vi "remove specific file path.vi"(8 "error in":errorcluster, 10 "Path":path, 11 "VI modification collection in":refnum<class "VI modification collection.lvclass">) -> (0 "error out":errorcluster, 3 "VI modification collection out":refnum<class "VI modification collection.lvclass">)   [LabVIEW 2013, in "VI modification collection.lvclass"]
uses:
  VI modification collection.lvclass
  VI modification collection.lvclass/VI modification collection.ctl
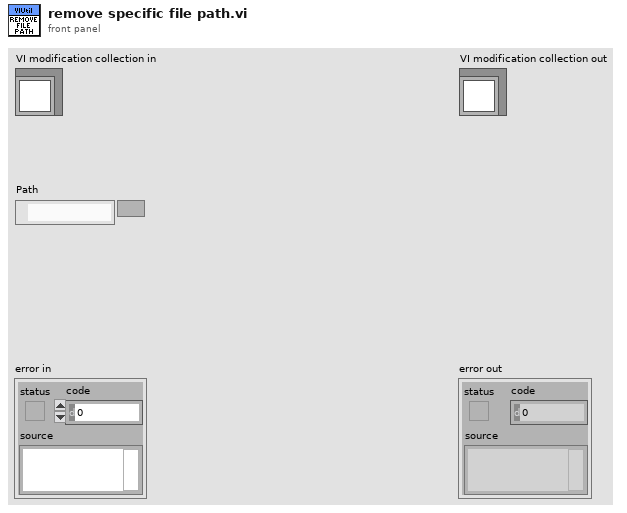
[diagram p1: front panel]
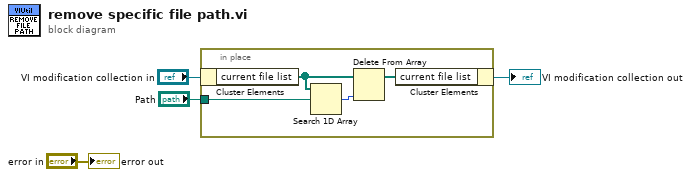
[diagram p0: block diagram]
diagram:
  n1 = in-place {
    in-place-border: "Path" -> [w8]
    n2 = in-place-cluster #1("VI modification collection in") -> ("current file list"=w7:path[])
    n3 = Search 1D Array(1D array=w7, element=w8) -> (index of element=w6:i32)  [unwired: 1 in]
    n4 = Delete From Array(array=w7, index=w6) -> (array with subset deleted=w5:path[])  [unwired: 1 in, 1 out]
    n5 = in-place-cluster #1("current file list"=w5) -> (→"VI modification collection out":refnum<class "VI modification collection.lvclass">)
  }
  "error out" <- "error in"
